vi "WAPIAerPosgrabReadPosition.vi"(3 "idx":i32, 9 "error in (no error)":errorcluster) -> (0 "pos":i32[](array[numeric]), 6 "error out":errorcluster)   [LabVIEW 2009]
uses:
  win50032.dll
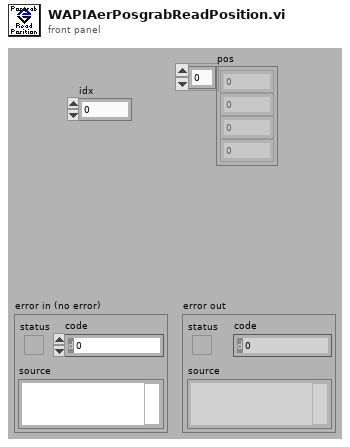
[diagram p1: front panel]
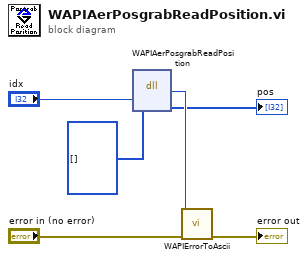
[diagram p0: block diagram]
diagram:
  n1 = dll-call lib="Win50032.dll" fn="WAPIAerPosgrabReadPosition"("idx"="idx", "pos"=i32[] []) -> ("return type"=w6:u32, "pos"=→"pos":i32[])  [unwired: 4 in, 2 out]
  n2 = call "WAPIErrorToAscii.vi"("error in (no error)"="error in (no error)", "error"=w6) -> ("error out"=→"error out":errorcluster)  [unwired: 8 in, 1 out]
